vi "Tanque_actual_labview.vi"() -> ()   [LabVIEW 2024]
uses:
  <vilib>/express/express arith-compare/Formula/XNode/ExpressFormulaBlockNode.xnode
panel:
  in  "Area (m^2)":dbl=2.0
  in  "Paro":bool
  in  "Alpha":dbl=10.0
  in  "a2":dbl=0.39999999999999997 min=0.0 max=1.05 step=0.05
  in  "a1":dbl=0.49999999999999994 min=0.0 max=1.05 step=0.05
  in  "k2":dbl=0.05 min=0.0 max=1.05 step=0.05
  out "Tanque":dbl(slide) scale=0.0..5.0
  in  "dt (s)":i64=10
  in  "h_t_1 (m)":dbl
  in  "k1":dbl=0.10000000000000002 min=0.0 max=1.05 step=0.05
  in  "Enum 2":enum16{"Lineal", "Rápida", "Isoporcentual"}(ring)
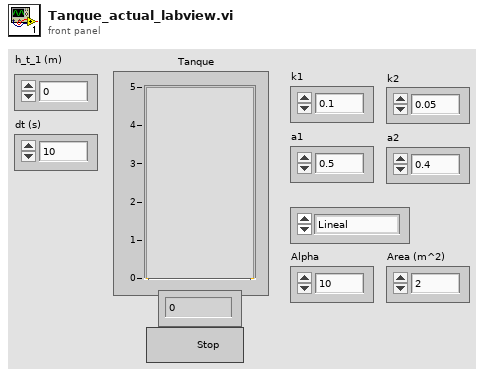
[diagram p1: front panel]
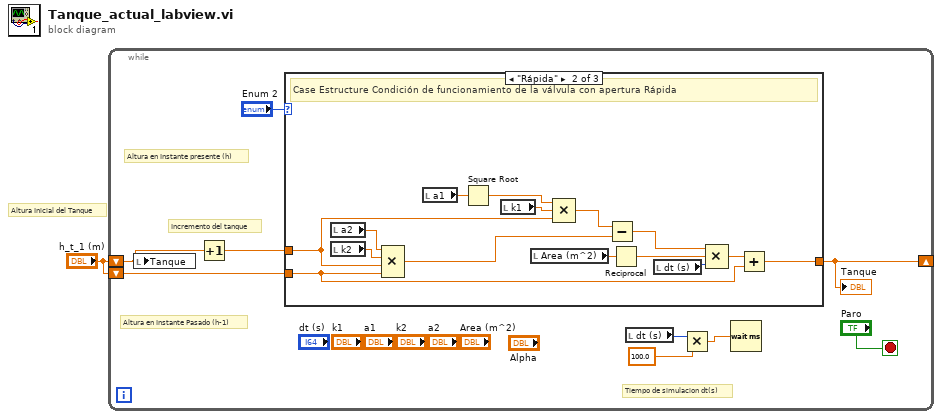
[diagram p0: block diagram]
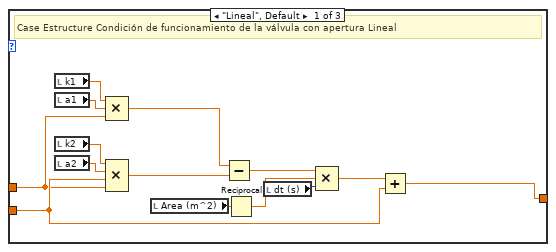
[diagram p2: hidden frame]
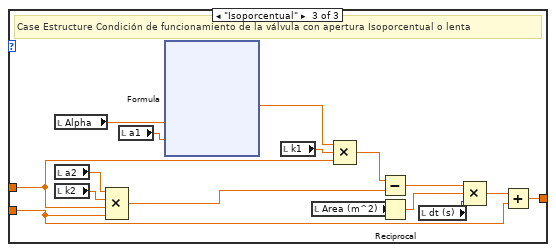
[diagram p3: hidden frame]
diagram:
  # "Altura Inicial del Tanque"
  n1 = while {
    shift-right: [w8] -> _
    shift-left: "h_t_1 (m)" -> [w5]
    shift-left: "h_t_1 (m)" -> [w9]
    stop <- "Paro" stop-if-true
    # "Tiempo de simulacion dt(s)"
    # "Altura en Instante presente (h)"
    # "Altura en Instante Pasado (h-1)"
    # "Incremento del tanque"
    n2 = local write "Tanque"(w5) -> ()
    n3 = Increment(x=w5) -> (x+1=w6:dbl)
    n4 = case shown="\"Rápida\"" "Enum 2" {
      tunnel: w6 -> [w11 w33 w40]
      tunnel: w9 -> [w13 w26 w46]
      tunnel: [w12 w25 w45] -> w8
      frame "Lineal", Default {
        # "Case Estructure Condición de funcionamiento de la válvula con apertura Lineal"
        n5 = local read "k1"() -> (w24:dbl)
        n6 = local read "a1"() -> (w23:dbl)
        n7 = local read "k2"() -> (w21:dbl)
        n8 = local read "a2"() -> (w20:dbl)
        n9 = Compound Arithmetic op=MULTIPLY(w24, w23, w11) -> (w22:dbl)
        n10 = Compound Arithmetic op=MULTIPLY(w21, w20, w13, w11) -> (w19:dbl)
        n11 = local read "Area (m^2)"() -> (w16:dbl)
        n12 = Subtract(x=w22, y=w19) -> (x-y=w18:dbl)
        n13 = Reciprocal(x=w16) -> (1/x=w15:dbl)
        n14 = local read "dt (s)"() -> (w17:i64)
        n15 = Compound Arithmetic op=MULTIPLY(w18, w15, w17) -> (w14:dbl)
        n16 = Add(x=w14, y=w13) -> (x+y=w12:dbl)
      }
      frame "Rápida" {
        # "Case Estructure Condición de funcionamiento de la válvula con apertura Rápida"
        n17 = local read "a2"() -> (w36:dbl)
        n18 = local read "k2"() -> (w35:dbl)
        n19 = Compound Arithmetic op=MULTIPLY(w36, w35, w33, w26) -> (w31:dbl)
        n20 = local read "a1"() -> (w39:dbl)
        n21 = Square Root(x=w39) -> (sqrt(x)=w38:dbl)
        n22 = local read "k1"() -> (w37:dbl)
        n23 = local read "Area (m^2)"() -> (w34:dbl)
        n24 = Compound Arithmetic op=MULTIPLY(w38, w37, w33) -> (w32:dbl)
        n25 = Subtract(x=w32, y=w31) -> (x-y=w30:dbl)
        n26 = Reciprocal(x=w34) -> (1/x=w29:dbl)
        n27 = local read "dt (s)"() -> (w28:i64)
        n28 = Compound Arithmetic op=MULTIPLY(w30, w29, w28) -> (w27:dbl)
        n29 = Add(x=w27, y=w26) -> (x+y=w25:dbl)
      }
      frame "Isoporcentual" {
        # "Case Estructure Condición de funcionamiento de la válvula con apertura Isoporcentual o lenta"
        n30 = local read "Alpha"() -> (w43:dbl)
        n31 = local read "a2"() -> (w49:dbl)
        n32 = local read "k2"() -> (w48:dbl)
        n33 = Compound Arithmetic op=MULTIPLY(w49, w48, w40, w46) -> (w54:dbl)
        n34 = local read "a1"() -> (w41:dbl)
        n35 = xnode "Formula"("X1"=w43, "X2"=w41) -> ("Result"=w44:dbl)  [unwired: 1 in, 1 out]
        n36 = local read "k1"() -> (w42:dbl)
        n37 = local read "Area (m^2)"() -> (w50:dbl)
        n38 = Compound Arithmetic op=MULTIPLY(w44, w42, w40) -> (w55:dbl)
        n39 = Subtract(x=w55, y=w54) -> (x-y=w53:dbl)
        n40 = Reciprocal(x=w50) -> (1/x=w52:dbl)
        n41 = local read "dt (s)"() -> (w47:i64)
        n42 = Compound Arithmetic op=MULTIPLY(w53, w52, w47) -> (w51:dbl)
        n43 = Add(x=w51, y=w46) -> (x+y=w45:dbl)
      }
    }
    "Tanque" <- w8
    n44 = local read "dt (s)"() -> (w3:i64)
    n45 = Multiply(x=w3, y=100.0) -> (x*y=w4:dbl)
    n46 = Wait (ms)(milliseconds to wait=w4) -> ()  [unwired: 1 out]
  }
